vi "Main.vi"   [LabVIEW 2019]
doc: "The myRIO Project template acquires acceleration data from the onboard accelerometer and displays the changes of acceleration values in a waveform chart."
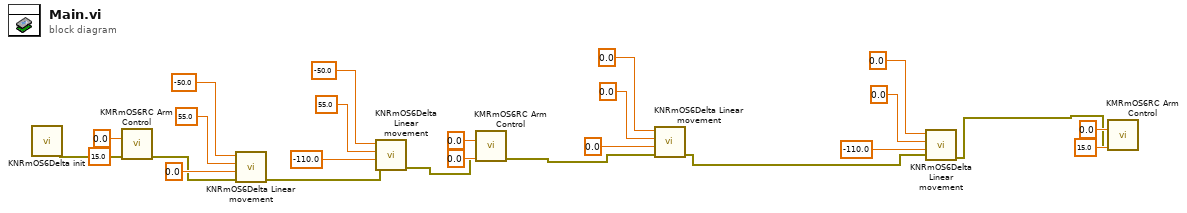
[diagram p0: block diagram]
diagram:
  n1 = call "KNRmOS6Delta init.vi"() -> ("error out"=w25:errorcluster)  [unwired: 11 in]
  n2 = call "KMRmOS6RC Arm Control.vi"("error in (no error)"=w25, "clip"=15.0, "turn"=0.0) -> ("error out"=w13:errorcluster)  [unwired: 6 in, 2 out]
  n3 = call "KNRmOS6Delta Linear movement.vi"("error in (no error)"=w13, "z0"=0.0, "y0"=55.0, "x0"=-50.0) -> ("error out"=w12:errorcluster)  [unwired: 7 in]
  n4 = call "KNRmOS6Delta Linear movement.vi"("error in (no error)"=w12, "z0"=-110.0, "y0"=55.0, "x0"=-50.0) -> ("error out"=w3:errorcluster)  [unwired: 7 in]
  n5 = call "KMRmOS6RC Arm Control.vi"("error in (no error)"=w3, "clip"=0.0, "turn"=0.0) -> ("error out"=w2:errorcluster)  [unwired: 6 in, 2 out]
  n6 = call "KNRmOS6Delta Linear movement.vi"("error in (no error)"=w2, "z0"=0.0, "y0"=0.0, "x0"=0.0) -> ("error out"=w1:errorcluster)  [unwired: 7 in]
  n7 = call "KNRmOS6Delta Linear movement.vi"("error in (no error)"=w1, "z0"=-110.0, "y0"=0.0, "x0"=0.0) -> ("error out"=w6:errorcluster)  [unwired: 7 in]
  n8 = call "KMRmOS6RC Arm Control.vi"("error in (no error)"=w6, "clip"=15.0, "turn"=0.0) -> ()  [unwired: 6 in, 3 out]
